vi "configure.vi"(8 "error in (no error)":errorcluster, 11 "lv-builder-l3 in":refnum<class "lv-builder-l3.lvclass">) -> (0 "error out":errorcluster, 3 "lv-builder-l3 out":refnum<class "lv-builder-l3.lvclass">)   [LabVIEW 2015, in "lv-builder-l3.lvlib" / "lv-builder-l3.lvclass"]
uses:
  lv-builder-l3.lvclass
  private/_controls/configuration_command.ctl
  lv-builder-l3.lvlib
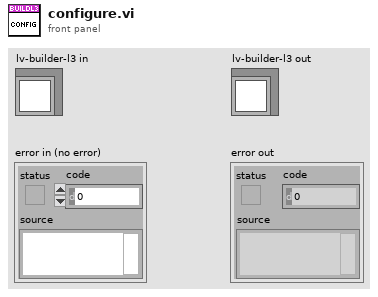
[diagram p1: front panel]
types:
  T1 = typedef "lv-builder-l3.lvlib/configuration_command.ctl" = enum16{"<config_command>", "read_config", "write_config", "<null>"}
  T2 = typedef "lv-builder-l3.lvlib/configuration.ctl" = cluster{"project_file":string, "l3_archive_file_path":string}
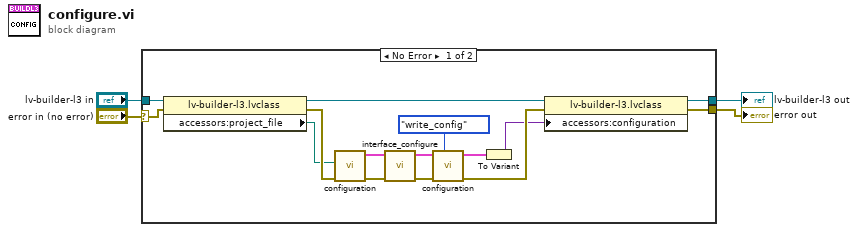
[diagram p0: block diagram]
diagram:
  n1 = case shown="No Error" "error in (no error)" {
    selector: "error in (no error)" -> [w8 w21]
    tunnel: "lv-builder-l3 in" -> [w14 w20]
    tunnel: [w9 w21] -> w1
    tunnel: [w12 w20] -> w3
    frame No Error {
      n2 = property class="lv-builder-l3.lvclass"(reference=w14, error in=w8) -> (reference out=w13:refnum<class "lv-builder-l3.lvclass">, error out=w7:errorcluster, "accessors:project_file"=w5:path)
      n3 = call "configuration.vi"("error in (no error)"=w7, "project_file"=w5) -> ("error out"=w16:errorcluster, "config out"=w19:T2)  [unwired: 8 in]
      n4 = call "interface_configure.vi"("error in (no error)"=w16, "config in"=w19) -> ("error out"=w17:errorcluster, "config out"=w18:T2)  [unwired: 8 in]
      n5 = call "configuration.vi"("command"=configuration_command."write_config", "error in (no error)"=w17, "config in"=w18) -> ("error out"=w10:errorcluster, "config out"=w11:T2)  [unwired: 7 in]
      n6 = To Variant(anything=w11) -> (Variant=w6:variant)
      n7 = property class="lv-builder-l3.lvclass"(reference=w13, error in=w10, "accessors:configuration"=w6) -> (reference out=w12:refnum<class "lv-builder-l3.lvclass">, error out=w9:errorcluster)
    }
    frame Error {
    }
  }
  "error out" <- w1
  "lv-builder-l3 out" <- w3
